vi "cm_Right Click Menu.vi"(7 "Display State In":T1={"Chan"=[], "First Drop?"=FALSE, "Notifier Name"="", "Refresh View"=FALSE, "Scale to Input Range"=FALSE, "Linear View"=FALSE, "Display"={"Current"=6618880, "Peak"=6618880}, "Property/Method"=enum."No Update", "Time Display Ref"=[]}, 8 "error in (no error)":errorcluster, 9 "Run Mode?":bool, 11 "MenuRef":refnum<k9>) -> (0 "error out":errorcluster)   [LabVIEW 2009, in "Channel Monitor [System].xctl"]
uses:
  Channel Monitor [System].xctl
  cm_Channel Monitor State.ctl
  TypeDef/cm_Property_Method.ctl
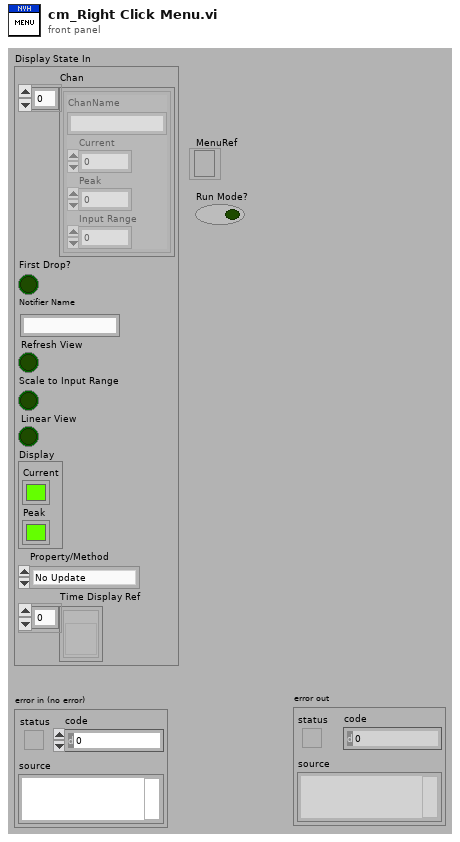
[diagram p1: front panel]
types:
  T1 = typedef "Channel Monitor [System].xctl/cm_Channel Monitor State.ctl" = cluster{"Chan":cluster{"ChanName":string, "Current":dbl, "Peak":dbl, "Input Range":dbl}[], "First Drop?":bool, "Notifier Name":string, "Refresh View":bool, "Scale to Input Range":bool, "Linear View":bool, "Display":cluster{"Current":u32, "Peak":u32}, "Property/Method":T2, "Time Display Ref":refnum<vi>[]}
  T2 = typedef "Channel Monitor [System].xctl/cm_Property_Method.ctl" = enum16{"No Update", "Color: Currrent", "Color: Peak", "Close Time Displays"}
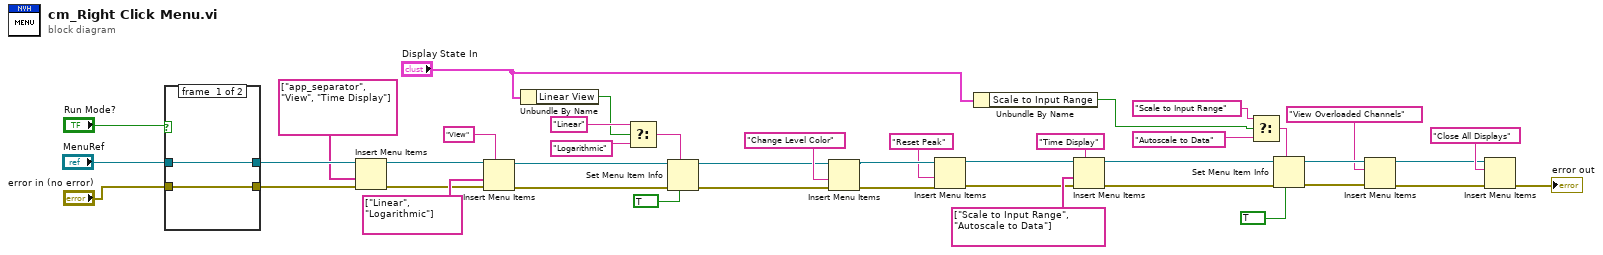
[diagram p0: block diagram]
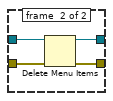
[diagram p2: hidden frame]
diagram:
  n1 = case shown="False" "Run Mode?" {
    tunnel: "MenuRef" -> [w44 w48]
    tunnel: [w44 w47] -> w29
    tunnel: "error in (no error)" -> [w43 w46]
    tunnel: [w43 w45] -> w14
    frame #0 {
    }
    frame #1 {
      n2 = Delete Menu Items(6:w46, 9:w48) -> (0:w45:errorcluster, 3:w47:refnum<k9>)  [unwired: 2 in]
    }
  }
  n3 = Insert Menu Items(6:w14, 7:string[] ["app_separator", "View", "Time Display"] ("item names"), 9:w29) -> (0:w13:errorcluster, 3:w32:refnum<k9>)  [unwired: 3 in, 1 out]
  n4 = Insert Menu Items(5:"View" ("menu tag"), 6:w13, 7:string[] ["Linear", "Logarithmic"] ("item tags"), 9:w32) -> (0:w12:errorcluster, 3:w35:refnum<k9>)  [unwired: 2 in, 1 out]
  n5 = Unbundle By Name("Display State In") -> ("Linear View"=w23:bool)
  n6 = Select(t="Linear", s=w23, f="Logarithmic") -> (s? t:f=w27:string)
  n7 = Set Menu Item Info(6:TRUE ("checked"), 7:w27, 8:w12, 11:w35) -> (0:w11:errorcluster, 3:w30:refnum<k9>)  [unwired: 3 in]
  n8 = Insert Menu Items(6:w11, 7:"Change Level Color", 9:w30) -> (0:w10:errorcluster, 3:w38:refnum<k9>)  [unwired: 3 in, 1 out]
  n9 = Insert Menu Items(6:w10, 7:"Reset Peak", 9:w38) -> (0:w9:errorcluster, 3:w39:refnum<k9>)  [unwired: 3 in, 1 out]
  n10 = Unbundle By Name("Display State In") -> ("Scale to Input Range"=w16:bool)
  n11 = Insert Menu Items(5:"Time Display" ("menu tag"), 6:w9, 7:string[] ["Scale to Input Range", "Autoscale to Data"] ("item tags"), 9:w39) -> (0:w8:errorcluster, 3:w41:refnum<k9>)  [unwired: 2 in, 1 out]
  n12 = Select(t="Scale to Input Range", s=w16, f="Autoscale to Data") -> (s? t:f=w18:string)
  n13 = Set Menu Item Info(6:TRUE ("checked"), 7:w18, 8:w8, 11:w41) -> (0:w5:errorcluster, 3:w2:refnum<k9>)  [unwired: 3 in]
  n14 = Insert Menu Items(6:w5, 8:"View Overloaded Channels", 9:w2) -> (0:w4:errorcluster, 3:w3:refnum<k9>)  [unwired: 3 in, 1 out]
  n15 = Insert Menu Items(6:w4, 8:"Close All Displays", 9:w3) -> (0:→"error out":errorcluster)  [unwired: 3 in, 2 out]
